vi "ThingWorxInit.vi"(9 "Properties":string[](array[string]), 11 "Input Info":T3={"ThingWorx Server Address"="52.202.159.58", "Port"="80", "Thing Name"="GenericEdge", "Application Key"="0aae8b5f-871a-4973-bdf2-199fabb27dcb", "Service Name"="UpdateValues"}) -> (0 "error out":errorcluster, 3 "Thing Info Out":T2)   [LabVIEW 2015]
uses:
  <vilib>/httpClient/ClientHandle.ctl
  <vilib>/httpClient/LabVIEWHTTPClient.lvlib
panel:
  in  "Thing Info Constant":T2
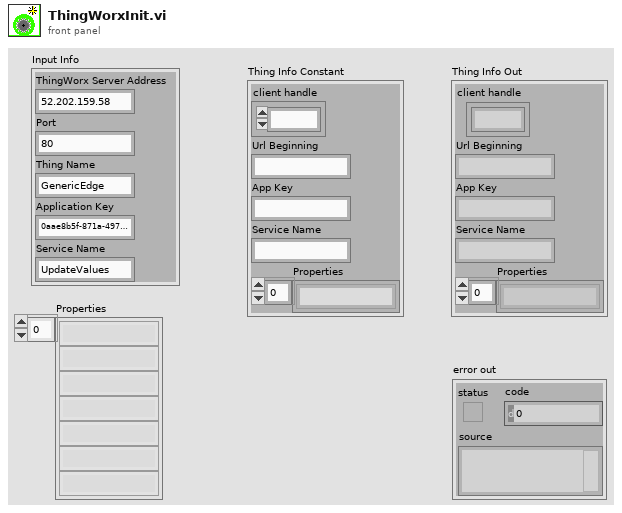
[diagram p1: front panel]
types:
  T1 = typedef "LabVIEWHTTPClient.lvlib/ClientHandle.ctl" = refnum<k1>
  T2 = cluster{"client handle":T1, "Url Beginning":string, "App Key":string, "Service Name":string, "Properties":string[]}
  T3 = cluster{"ThingWorx Server Address":string, "Port":string, "Thing Name":string, "Application Key":string, "Service Name":string}
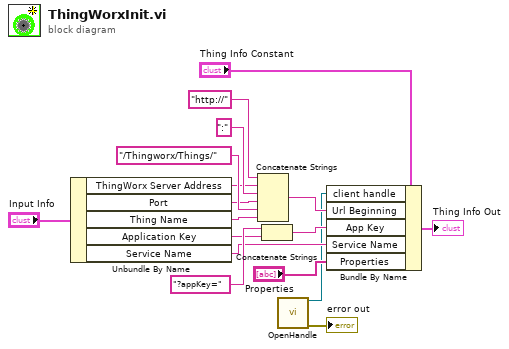
[diagram p0: block diagram]
diagram:
  n1 = Unbundle By Name("Input Info") -> ("ThingWorx Server Address"=w12:string, "Port"=w11:string, "Thing Name"=w10:string, "Application Key"=w9:string, "Service Name"=w6:string)
  n2 = Concatenate Strings("http://" ("url"), w12, ":" ("url"), w11, "/Thingworx/Things/" ("url"), w10) -> (w8:string)
  n3 = Concatenate Strings("?appKey=" ("url"), w9) -> (w7:string)
  n4 = call <vilib>:"OpenHandle.vi"() -> ("client handle out"=w2:T1, "error out"=→"error out":errorcluster)  [unwired: 14 in]
  n5 = Bundle By Name(cluster="Thing Info Constant", "client handle"=w2, "Url Beginning"=w8, "App Key"=w7, "Service Name"=w6, "Properties"="Properties") -> (→"Thing Info Out":T2)
